vi "CRYReport CheckActiveX.vi"(9 "pVIRef":refnum<vi>, 11 "pApplication":refnum<vi>) -> ()   [LabVIEW 2013]
uses:
  CRYMainGlobal.vi
panel:
  in  "TXButtonBar":refnum<k7>(container)
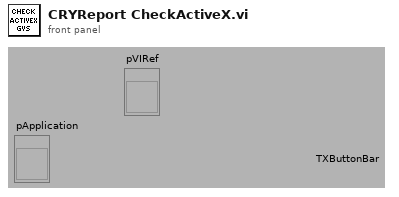
[diagram p1: front panel]
types:
  T1 = enum16{"open", "open or create", "create or replace", "create", "open (read only)"}
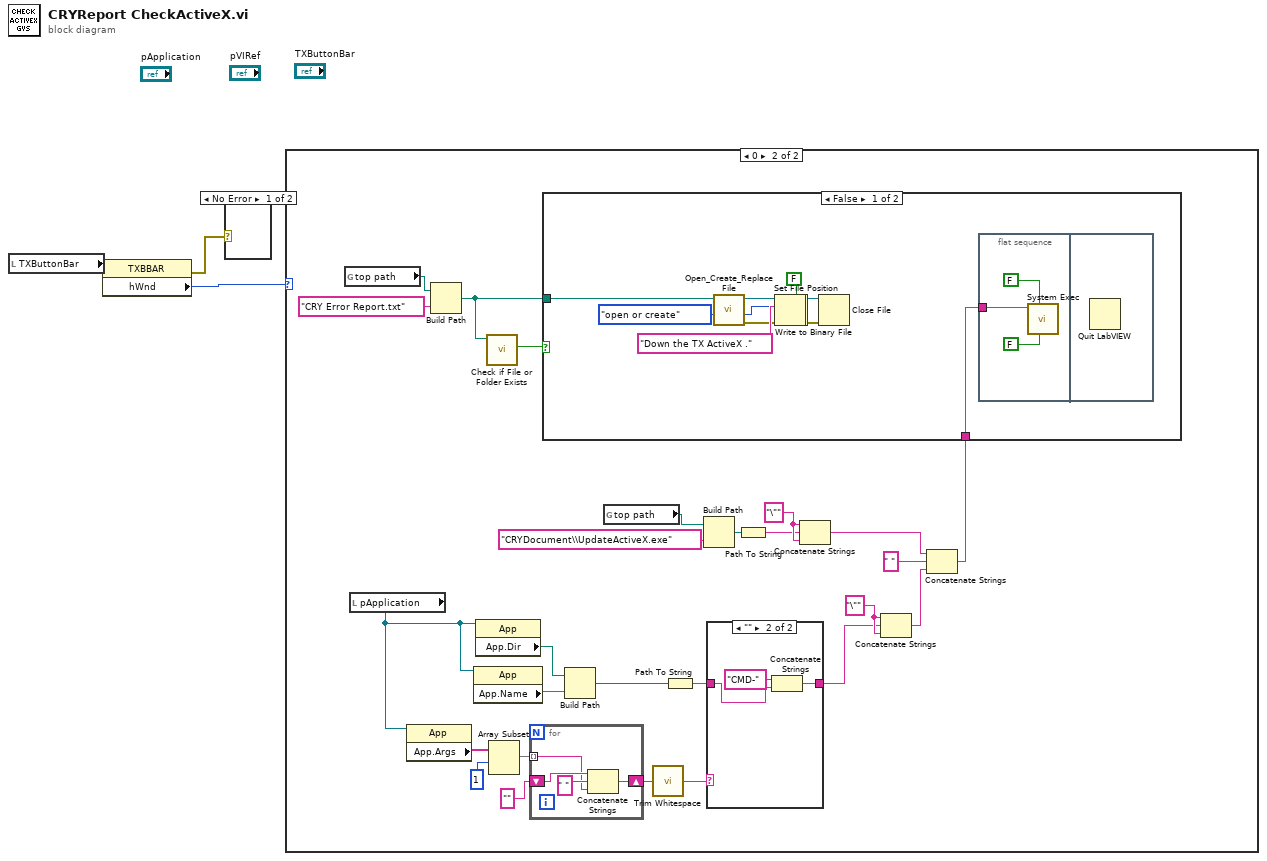
[diagram p0: block diagram]
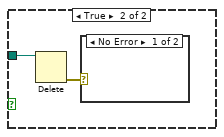
[diagram p4: hidden frame]
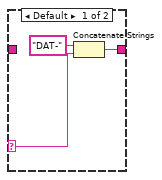
[diagram p6: hidden frame]
diagram:
  n1 = local read "TXButtonBar"() -> (w3:refnum<k7>)
  n2 = property class="TXBBAR"(reference=w3) -> (error out=w1:errorcluster, "hWnd"=w2:i32)  [unwired: 1 in, 1 out]
  n3 = case shown="No Error" w1 {
    frame No Error {
    }
    frame Error {
    }
  }
  n4 = case shown="0" w2 {
    frame Default {
    }
    frame 0 {
      w19 = "\"" ("string")
      w24 = "\"" ("string")
      n5 = global read "CRYMainGlobal.vi" "top path"() -> (w6:path)
      n6 = local read "pApplication"() -> (w16:refnum<vi>)
      n7 = property class="App"(reference=w16) -> ("App.Args"=w21:string[])  [unwired: 1 in, 2 out]
      n8 = Build Path(base path=w6, name or relative path="CRY Error Report.txt") -> (appended path=w8:path)
      n9 = property class="App"(reference=w16) -> ("App.Name"=w15:string)  [unwired: 1 in, 2 out]
      n10 = property class="App"(reference=w16) -> ("App.Dir"=w17:path)  [unwired: 1 in, 2 out]
      n11 = call <vilib>:"Check if File or Folder Exists.vi"("path"=w8) -> ("file or folder exists?"=w9:bool)  [unwired: 8 in, 2 out]
      n12 = Array Subset(array=w21, index=1 ("length")) -> (w22:string[])  [unwired: 1 in]
      n13 = for {
        tunnel: w22 -> [w53] mode=indexing
        shift-right: [w55] -> w28
        shift-left: "" -> [w56]
        n14 = Concatenate Strings(w56, " " ("string"), w53) -> (w55:string)
      }
      n15 = Build Path(base path=w17, name or relative path=w15) -> (appended path=w4:path)
      n16 = global read "CRYMainGlobal.vi" "top path"() -> (w10:path)
      n17 = call <vilib>:"Trim Whitespace.vi"("string"=w28) -> ("trimmed string"=w14:string)  [unwired: 1 in]
      n18 = Path To String(path=w4) -> (string=w13:string)
      n19 = Build Path(base path=w10, name or relative path="CRYDocument\\UpdateActiveX.exe") -> (appended path=w29:path)
      n20 = case shown="\"\"" w14 {
        selector: w14 -> [w47 _]
        tunnel: w13 -> [_ w50]
        tunnel: [w49 w52] -> w12
        frame Default {
          n21 = Concatenate Strings("DAT-" ("string"), w47) -> (w49:string)
        }
        frame "" {
          n22 = Concatenate Strings("CMD-" ("string"), w50) -> (w52:string)
        }
      }
      n23 = Path To String(path=w29) -> (string=w11:string)
      n24 = Concatenate Strings(w24, w11, w24) -> (w23:string)
      n25 = Concatenate Strings(w19, w12, w19) -> (w18:string)
      n26 = Concatenate Strings(w23, " " ("string"), w18) -> (w5:string)
      n27 = case shown="False" w9 {
        tunnel: w8 -> [w31 w46]
        tunnel: w5 -> [w30 _]
        frame False {
          n28 = call <vilib>:"Open_Create_Replace File.vi"("function (open:0)"=T1."open or create", "file path"=w31) -> ("error out"=w33:errorcluster, "file size (bytes)"=w35:i32, "refnum"=w34:refnum<file>)  [unwired: 6 in, 1 out]
          n29 = Set File Position(offset (in bytes) (0)=w35, refnum=w34, error in=w33) -> (refnum out=w38:refnum<file>, error out=w39:errorcluster)  [unwired: 1 in]
          n30 = Write to Binary File(file (use dialog)=w38, data="Down the TX ActiveX .", error in=w39, 5:FALSE ("prepend array or string size? (T)")) -> (refnum out=w37:refnum<file>, error out=w36:errorcluster)  [unwired: 2 in, 1 out]
          n31 = Close File(refnum=w37, error in=w36) -> ()  [unwired: 2 out]
          n32 = flat-sequence {
            tunnel: w30 -> [w42]
            frame #0 {
              n33 = call <vilib>:"System Exec.vi"("run minimized? (F)"=FALSE, "wait until completion? (T)"=FALSE, "command line"=w42) -> ()  [unwired: 3 in, 6 out]
            }
            frame #1 {
              n34 = Quit LabVIEW() -> ()  [unwired: 1 in]
            }
          }
        }
        frame True {
          n35 = Delete(path (use dialog)=w46) -> (error out=w45:errorcluster)  [unwired: 4 in, 2 out]
          n36 = case shown="No Error" w45 {
            frame No Error {
            }
            frame Error {
            }
          }
        }
      }
    }
  }
